vi "Single Channel Read.vi"(8 "error in (no error)":errorcluster, 10 "Numeric":i8 min=0 max=20, 11 "VISA resource name":refnum<visa-resource-name>) -> (0 "error out":errorcluster, 1 "concatenated string":string, 2 "number":dbl, 3 "VISA resource name out":refnum<visa-resource-name>, 5 "read buffer":string)   [LabVIEW 2013, in "Fluke 2625A.lvlib"]
uses:
  <instrlib>/Fluke 2625A/Fluke 2625A.lvlib
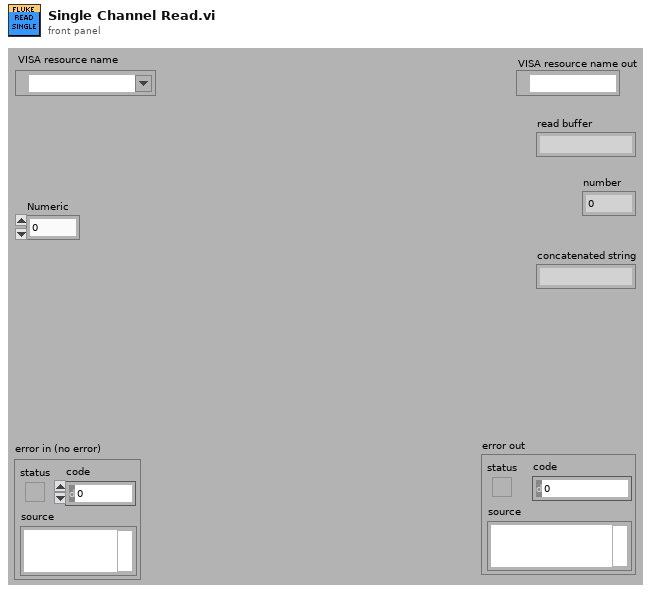
[diagram p1: front panel]
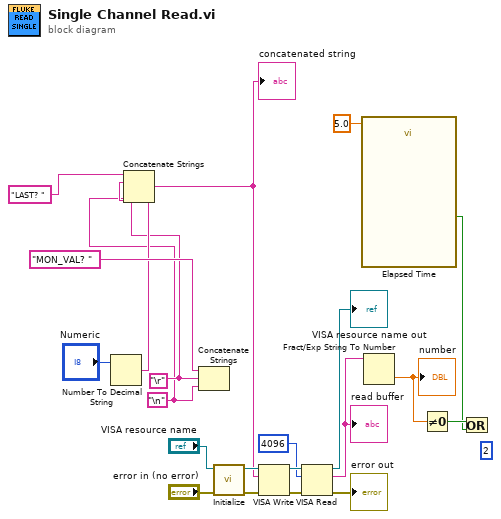
[diagram p0: block diagram]
diagram:
  w1 = "\n"
  (unwired) 2
  w2 = "\r"
  n1 = Number To Decimal String(number="Numeric") -> (decimal integer string=w4:string)  [unwired: 1 in]
  n2 = Concatenate Strings("LAST? " ("string"), w4, w2, w1) -> (w3:string)
  "concatenated string" <- w3
  n3 = Concatenate Strings("MON_VAL? " ("string"), w2, w1) -> ()  [unwired: 1 out]
  n4 = call <instrlib>:"Initialize.vi"("error In"="error in (no error)", "VISA resource name"="VISA resource name") -> ("error out"=w18:errorcluster, "VISA resource name out"=w19:refnum<visa-resource-name>)  [unwired: 7 in, 1 out]
  n5 = VISA Write(VISA resource name=w19, write buffer=w3, error in (no error)=w18) -> (VISA resource name out=w16:refnum<visa-resource-name>, error out=w14:errorcluster)  [unwired: 1 out]
  n6 = VISA Read(VISA resource name=w16, byte count=u32 4096, error in (no error)=w14) -> (VISA resource name out=→"VISA resource name out":refnum<visa-resource-name>, read buffer=w12:string, error out=→"error out":errorcluster)  [unwired: 1 out]
  "read buffer" <- w12
  n7 = call "Elapsed Time"("Time Target (s)"=5.0) -> ("Time has Elapsed"=w7:bool)  [unwired: 11 in, 7 out]
  n8 = Fract/Exp String To Number(string=w12) -> (number=w10:dbl)  [unwired: 3 in, 1 out]
  "number" <- w10
  n9 = Not Equal To 0?(x=w10) -> (x != 0?=w8:bool)
  n10 = Or(x=w8, y=w7) -> ()  [unwired: 1 out]
